vi "Load State Machine.vi"   [LabVIEW 2013]
uses:
  typedefs/fg_typedef.ctl
  typedefs/State Machine/singleUseSubstate.ctl
  <vilib>/Rock Robotics/WPI/Solenoid/WPI_SolenoidValue.ctl
  typedefs/DevRef Type.ctl
  typedefs/State Machine/subStates.ctl
  <vilib>/Rock Robotics/WPI/Solenoid/WPI_SolenoidGetEnum.vi
panel:
  # "A State Machine to Handle Loading for Either High or Low Goal Shots"
types:
  T1 = typedef "fg_typedef.ctl" = enum16{"Get", "Set"}
  T2 = typedef "DevRef Type.ctl" = enum16{"Shooter Solenoid", "Latch Solenoid", "Right Up Sensor", "Right Down Sensor", "Hold Sensor", "2 Ball Switch", "Arm Encoder"}
  T3 = typedef "WPI_SolenoidValue.ctl" = enum16{"Off", "On", "Forward", "Reverse"}
  T4 = typedef "singleUseSubstate.ctl" = enum16{"null", "wait", "shift high", "shift low", "extend shooter", "retract shooter", "latch", "unlatch", "end"}
  T5 = typedef "subStates.ctl" = enum16{"null", "wait", "driver control", "auto", "manual override", "hold position", "rotate", "pickup", "pass", "recover pass", "load", "goto shoot", "shoot high goal", "shoot low goal", "cancel arm", "cancel shooter", "end", "test"}
  T6 = typedef "WPI_SolenoidDevRef.ctl" = cluster{"DevStatus":errorcluster, "Solenoid Module":T7, "Forward Solenoid Channel":T8, "Reverse Solenoid Channel":T8}
  T7 = typedef "FPGA_TypedefSolenoidModule.ctl" = enum16{"Solenoid Module 1", "Solenoid Module 2"}
  T8 = typedef "WPI_SolenoidChannel.ctl" = enum8{"Solenoid 1", "Solenoid 2", "Solenoid 3", "Solenoid 4", "Solenoid 5", "Solenoid 6", "Solenoid 7", "Solenoid 8", "Invalid"}
  T9 = typedef "WPI_DigitalInputDevRef.ctl" = cluster{"DevStatus":errorcluster, "DIO Channel":T10, "Digital Module":T11}
  T10 = typedef "FPGA_DIOChannel.ctl" = enum8{"DIO 1", "DIO 2", "DIO 3", "DIO 4", "DIO 5", "DIO 6", "DIO 7", "DIO 8", "DIO 9", "DIO 10", "DIO 11", "DIO 12", "DIO 13", "DIO 14", "Invalid"}
  T11 = typedef "FPGA_TypedefDigitalModule.ctl" = enum16{"Digital Module 1", "Digital Module 2"}
  T12 = typedef "WPI_EncoderDevRef.ctl" = cluster{"DevStatus":errorcluster, "EncoderIndex":T13, "CounterIndex":T14, "DistancePerCount":dbl, "Decoding Type":T15}
  T13 = typedef "FPGA_EncoderIdx.ctl" = enum8{"Enc 0", "Enc 1", "Enc 2", "Enc 3", "Invalid"}
  T14 = typedef "FPGA_CounterCtrSystemIndex.ctl" = enum8{"Ctr 0", "Ctr 1", "Ctr 2", "Ctr 3", "Ctr 4", "Ctr 5", "Ctr 6", "Ctr 7", "Invalid"}
  T15 = typedef "WPI_EncoderType.ctl" = enum16{"1x", "2x", "4x"}
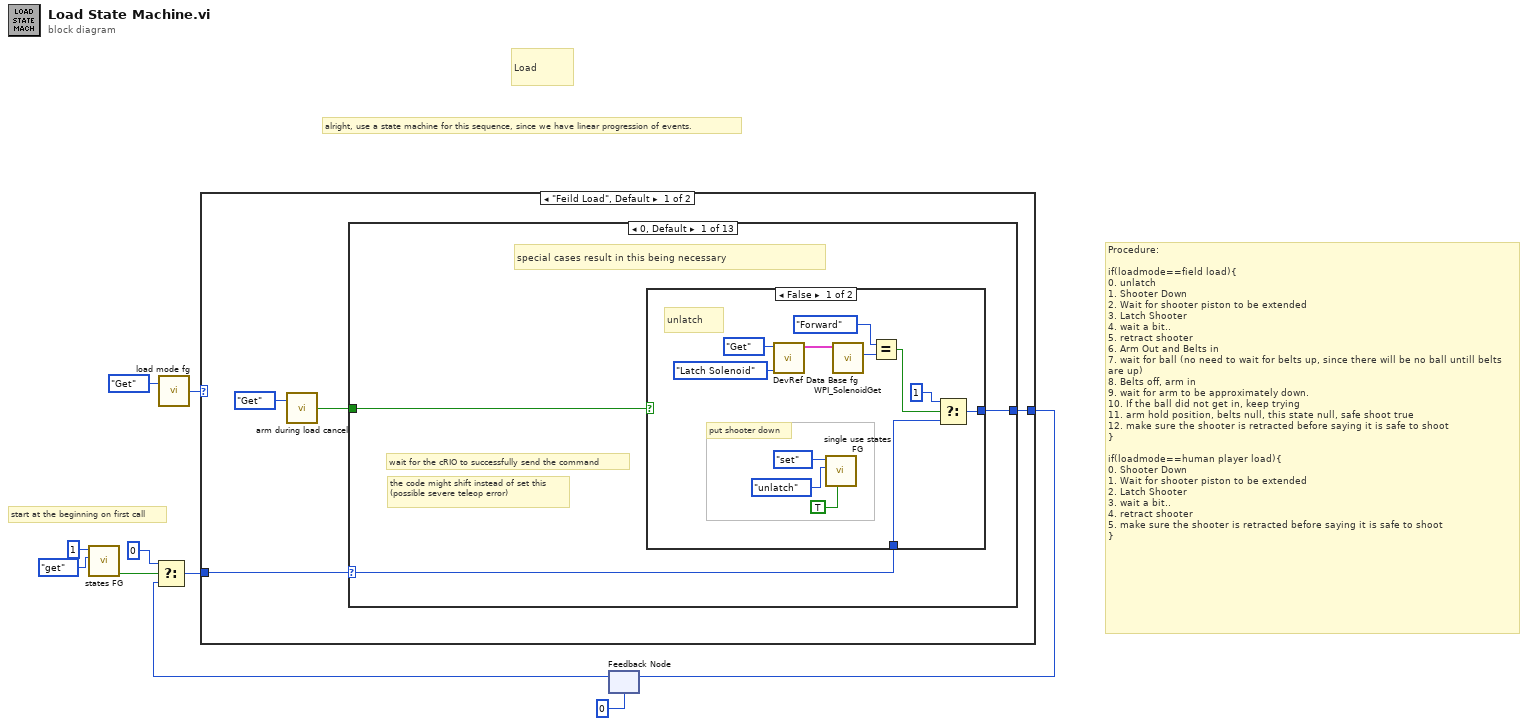
[diagram p0: block diagram]
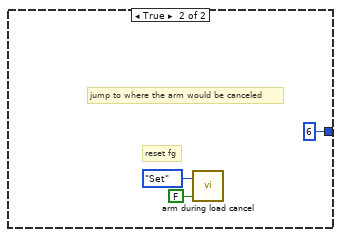
[diagram p2: hidden frame]
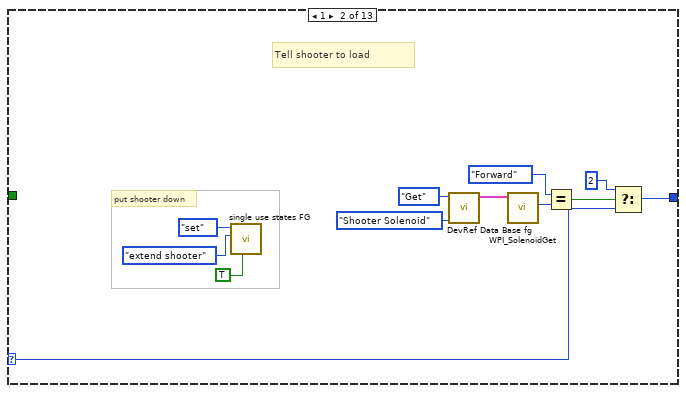
[diagram p3: hidden frame]
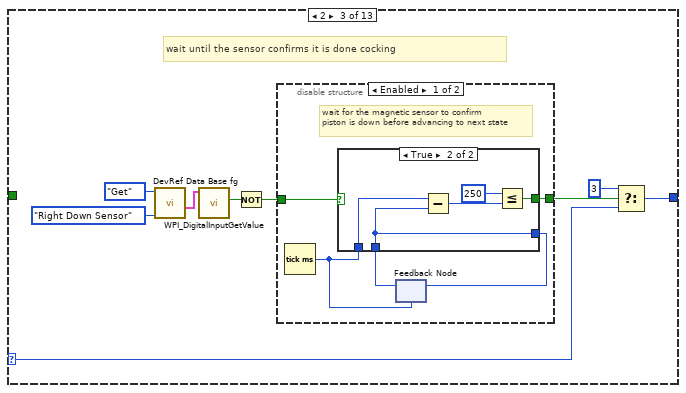
[diagram p4: hidden frame]
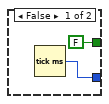
[diagram p5: hidden frame]
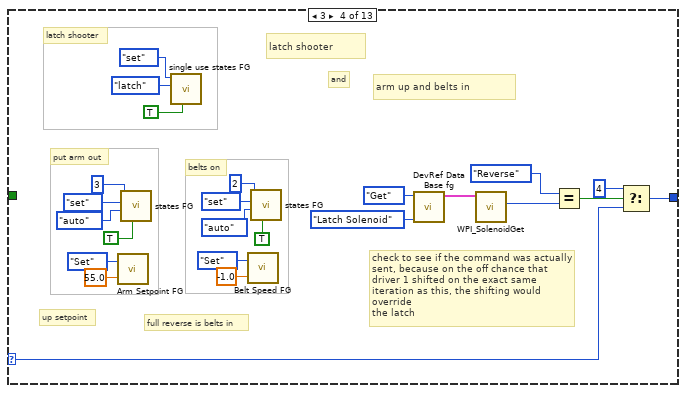
[diagram p7: hidden frame]
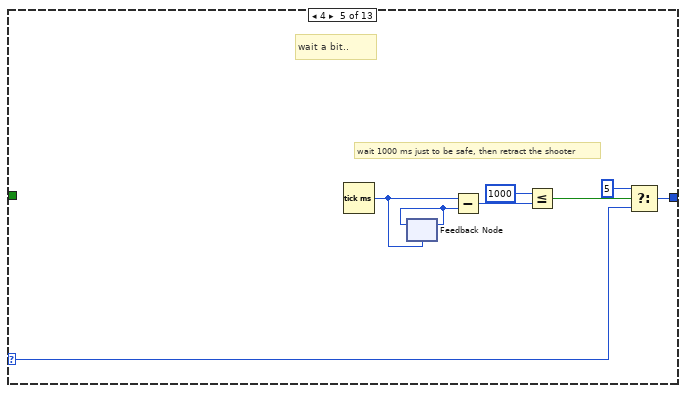
[diagram p8: hidden frame]
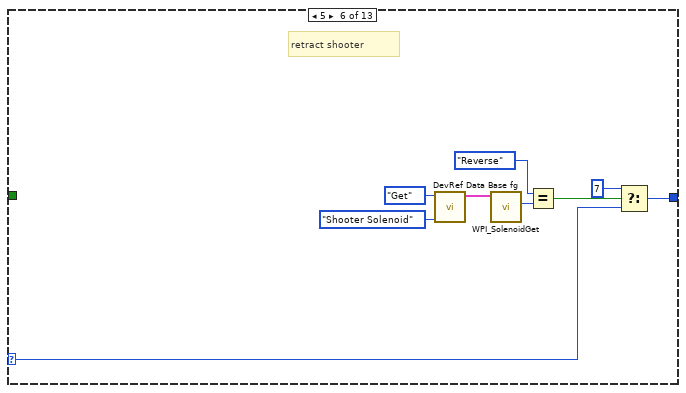
[diagram p9: hidden frame]
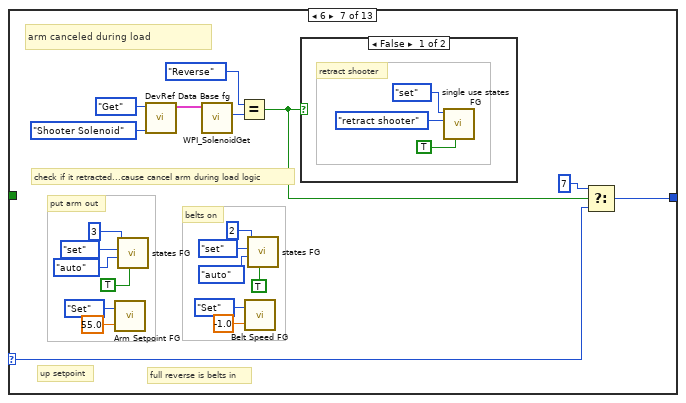
[diagram p10: hidden frame]
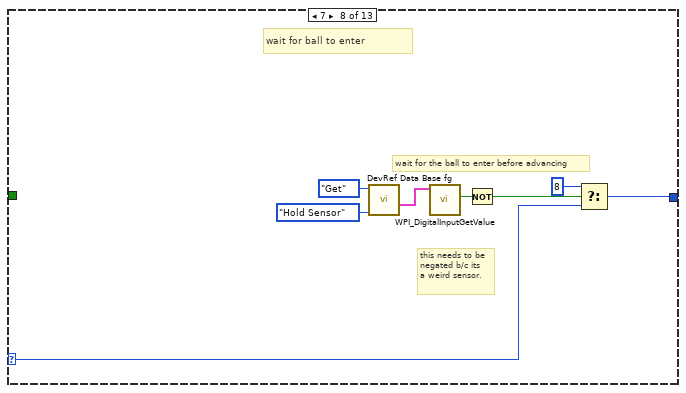
[diagram p12: hidden frame]
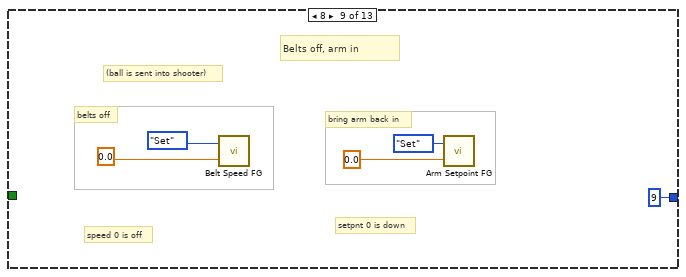
[diagram p13: hidden frame]
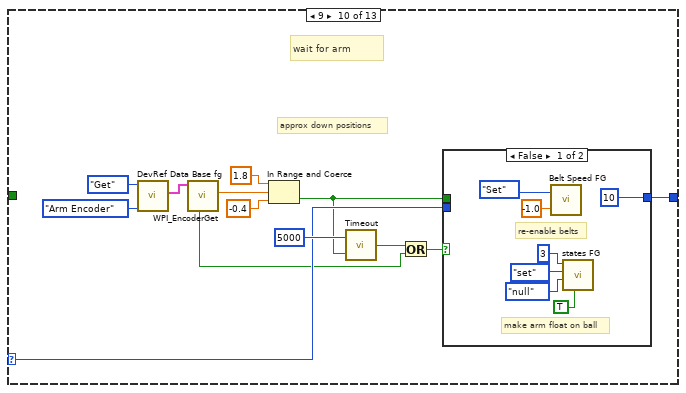
[diagram p14: hidden frame]
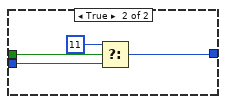
[diagram p15: hidden frame]
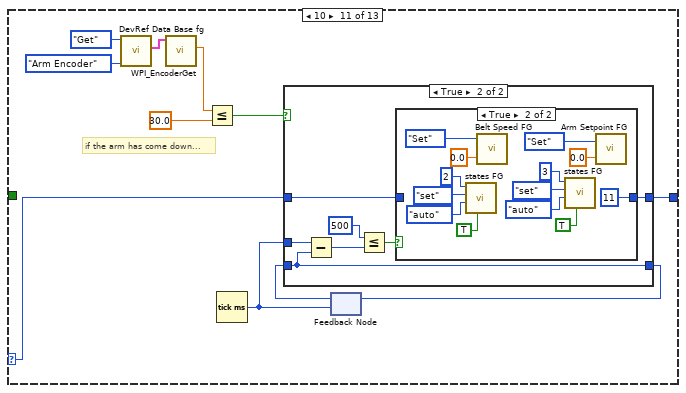
[diagram p16: hidden frame]
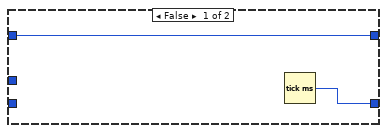
[diagram p17: hidden frame]
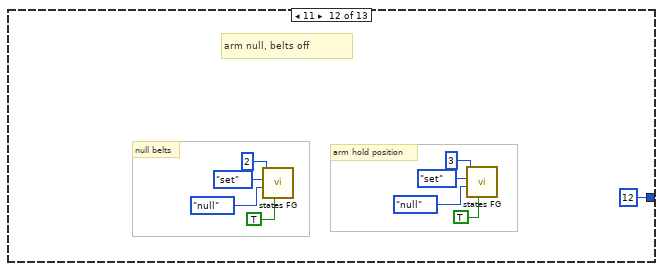
[diagram p19: hidden frame]
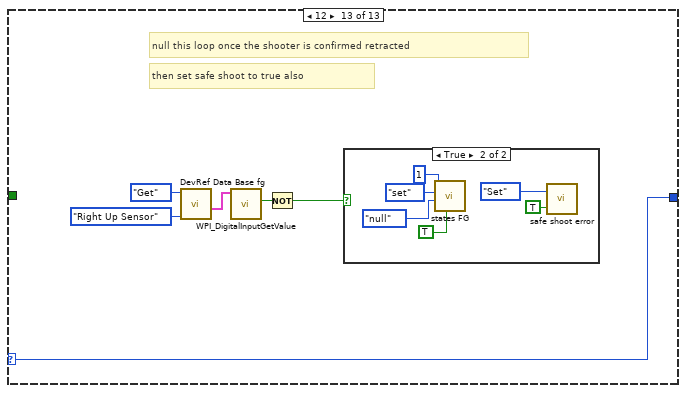
[diagram p20: hidden frame]
diagram:
  # "start at the beginning on first call"
  # "Load"
  # "Procedure: \n\nif(loadmode==field load){\n0. unlatch\n1. Shooter Down \n2. Wait for shooter piston to be extended\n3. Latch Shooter\n4. wait a bit..\n5. retract shooter\n6. Arm Out and Belts in\n7. wait for ball (no need to wait for belts up, since there will be no ball untill belts are up)\n8. Belts off, arm in\n9. wait for arm to be approximately down.\n10. If the ball did not get in, keep trying\n11. arm hold position, belts null, this state null, safe shoot true\n12. make sure the shooter is retracted before saying it is safe to shoot\n}\n\nif(loadmode==human player load){\n0. Shooter Down \n1. Wait for shooter piston to be extended\n2. Latch Shooter\n3. wait a bit..\n4. retract shooter\n5. make sure the shooter is retracted before saying it is safe to shoot\n}"
  # "alright, use a state machine for this sequence, since we have linear progression of events."
  n1 = call "states FG.vi"("menu (get)"=enum16{"set", "get"}."get", "Loop ID"=1) -> ("first call?"=w3:bool)  [unwired: 6 in, 3 out]
  n2 = call "load mode fg.vi"("Menu"=fg_typedef."Get") -> ("Load Mode"=w2:enum16{"Feild Load", "Human Player Load"})  [unwired: 1 in]
  n3 = feedback #1(u8 0) -> (w4:u8)
  n4 = Select(t=u8 0, s=w3, f=w4) -> (s? t:f=w6:u8)
  n5 = case shown="\"Feild Load\", Default" w2 {
    tunnel: [w14 w225] -> w9
    tunnel: w6 -> [w13 w224]
    frame "Feild Load", Default {
      n6 = call "arm during load cancel.vi"("Mode"=enum16{"Get", "Set", "Teleop Set"}."Get") -> ("Arm Canceled During Load"=w11:bool)  [unwired: 1 in]
      n7 = case shown="0, Default" w13 {
        selector: w13 -> [w16 w33 w51 w86 w92 w107 w120 w137 _ w149 w169 _ w217]
        tunnel: [w17 w34 w50 w87 w94 w106 w121 w136 u8 9 ("t") w150 w171 u8 12 ("t") w217] -> w14
        tunnel: w11 -> [w15 _ _ _ _ _ _ _ _ _ _ _ _]
        frame 0, Default {
          # "the code might shift instead of set this\n(possible severe teleop error)"
          # "special cases result in this being necessary"
          # "wait for the cRIO to successfully send the command"
          n8 = case shown="False" w15 {
            tunnel: [w26 u8 6 ("t")] -> w17
            tunnel: w16 -> [w25 _]
            frame False {
              # "unlatch"
              # "put shooter down"
              n9 = call "DevRef Data Base fg.vi"("DevRef to Get"=DevRef_Type."Latch Solenoid", "Menu"=fg_typedef."Get") -> ("Selected Solenoid"=w24:T6)  [unwired: 2 in, 5 out]
              n10 = call "single use states FG.vi"("exit in"=TRUE, "substate"=singleUseSubstate."unlatch", "menu (get)"=enum16{"set", "get"}."set") -> ()  [unwired: 5 in, 4 out]
              n11 = call-poly <vilib>:"WPI_SolenoidGet.vi"("SolenoidDevRef"=w24) -> ("Value"=w23:T3)  [unwired: 8 in, 2 out]
              n12 = Equal?(x=WPI_SolenoidValue."Forward", y=w23) -> (x = y?=w21:bool)
              n13 = Select(t=u8 1, s=w21, f=w25) -> (s? t:f=w26:u8)
            }
            frame True {
              # "reset fg"
              # "jump to where the arm would be canceled"
              n14 = call "arm during load cancel.vi"("Arm Canceled During Load?"=FALSE, "Mode"=enum16{"Get", "Set", "Teleop Set"}."Set") -> ()  [unwired: 1 out]
            }
          }
        }
        frame 1 {
          # "Tell shooter to load"
          # "put shooter down"
          n15 = call "single use states FG.vi"("exit in"=TRUE, "substate"=singleUseSubstate."extend shooter", "menu (get)"=enum16{"set", "get"}."set") -> ()  [unwired: 5 in, 4 out]
          n16 = call "DevRef Data Base fg.vi"("DevRef to Get"=DevRef_Type."Shooter Solenoid", "Menu"=fg_typedef."Get") -> ("Selected Solenoid"=w41:T6)  [unwired: 2 in, 5 out]
          n17 = call-poly <vilib>:"WPI_SolenoidGet.vi"("SolenoidDevRef"=w41) -> ("Value"=w40:T3)  [unwired: 8 in, 2 out]
          n18 = Equal?(x=WPI_SolenoidValue."Forward", y=w40) -> (x = y?=w38:bool)
          n19 = Select(t=u8 2, s=w38, f=w33) -> (s? t:f=w34:u8)
        }
        frame 2 {
          # "wait until the sensor confirms it is done cocking"
          n20 = call "DevRef Data Base fg.vi"("DevRef to Get"=DevRef_Type."Right Down Sensor", "Menu"=fg_typedef."Get") -> ("Selected Sensor"=w52:T9)  [unwired: 2 in, 5 out]
          n21 = call <vilib>:"WPI_DigitalInputGetValue.vi"("DigitalInputDevRef"=w52) -> ("Value"=w53:bool)  [unwired: 8 in, 2 out]
          n22 = Not(x=w53) -> (.not. x?=w46:bool)
          n23 = disable-structure shown="Enabled" {
            disable-tunnel: w46 -> [w58 w66]
            disable-tunnel: [w54 w66] -> w45
            frame Enabled {
              # "wait for the magnetic sensor to confirm \npiston is down before advancing to next state"
              n24 = Tick Count (ms)() -> (millisecond timer value=w57:u32)
              n25 = feedback #2(w57) -> (w55:u32)
              n26 = case shown="True" w58 {
                tunnel: w57 -> [_ w63]
                tunnel: [w60 w61] -> w56
                tunnel: w55 -> [_ w61]
                tunnel: [FALSE w62] -> w54
                frame False {
                  n27 = Tick Count (ms)() -> (millisecond timer value=w60:u32)
                }
                frame True {
                  n28 = Subtract(x=w63, y=w61) -> (x-y=w65:u32)
                  n29 = Less Or Equal?(x=u32 250, y=w65) -> (x <= y?=w62:bool)
                }
              }
              n30 = feedback-in #2(w56) -> ()
            }
            frame Disabled {
            }
          }
          n31 = Select(t=u8 3, s=w45, f=w51) -> (s? t:f=w50:u8)
        }
        frame 3 {
          # "latch shooter"
          # "full reverse is belts in"
          # "belts on"
          # "up setpoint"
          # "put arm out"
          # "and"
          # "arm up and belts in"
          # "check to see if the command was actually\nsent, because on the off chance that\ndriver 1 shifted on the exact same\niteration as this, the shifting would override\nthe latch"
          # "latch shooter"
          n32 = call "Arm Setpoint FG.vi"("Setpoint In"=55.0, "Menu"=fg_typedef."Set") -> ()  [unwired: 1 out]
          n33 = call "states FG.vi"("exit in"=TRUE, "subState in"=subStates."auto", "menu (get)"=enum16{"set", "get"}."set", "Loop ID"=3) -> ()  [unwired: 4 in, 4 out]
          n34 = call "single use states FG.vi"("exit in"=TRUE, "substate"=singleUseSubstate."latch", "menu (get)"=enum16{"set", "get"}."set") -> ()  [unwired: 5 in, 4 out]
          n35 = call "Belt Speed FG.vi"("Speed In"=-1.0 ("Setpoint In"), "Menu"=fg_typedef."Set") -> ()  [unwired: 1 out]
          n36 = call "states FG.vi"("exit in"=TRUE, "subState in"=subStates."auto", "menu (get)"=enum16{"set", "get"}."set", "Loop ID"=2) -> ()  [unwired: 4 in, 4 out]
          n37 = call "DevRef Data Base fg.vi"("DevRef to Get"=DevRef_Type."Latch Solenoid", "Menu"=fg_typedef."Get") -> ("Selected Solenoid"=w85:T6)  [unwired: 2 in, 5 out]
          n38 = call-poly <vilib>:"WPI_SolenoidGet.vi"("SolenoidDevRef"=w85) -> ("Value"=w84:T3)  [unwired: 8 in, 2 out]
          n39 = Equal?(x=WPI_SolenoidValue."Reverse" ("Value"), y=w84) -> (x = y?=w82:bool)
          n40 = Select(t=u8 4, s=w82, f=w86) -> (s? t:f=w87:u8)
        }
        frame 4 {
          # "wait a bit.."
          # "wait 1000 ms just to be safe, then retract the shooter"
          n41 = Tick Count (ms)() -> (millisecond timer value=w96:u32)
          n42 = feedback #3(w96) -> (w97:u32)
          n43 = feedback-in #3(w97) -> ()
          n44 = Subtract(x=w96, y=w97) -> (x-y=w95:u32)
          n45 = Less Or Equal?(x=u32 1000, y=w95) -> (x <= y?=w93:bool)
          n46 = Select(t=u8 5, s=w93, f=w92) -> (s? t:f=w94:u8)
        }
        frame 5 {
          # "retract shooter"
          n47 = call "DevRef Data Base fg.vi"("DevRef to Get"=DevRef_Type."Shooter Solenoid", "Menu"=fg_typedef."Get") -> ("Selected Solenoid"=w105:T6)  [unwired: 2 in, 5 out]
          n48 = call-poly <vilib>:"WPI_SolenoidGet.vi"("SolenoidDevRef"=w105) -> ("Value"=w104:T3)  [unwired: 8 in, 2 out]
          n49 = Equal?(x=WPI_SolenoidValue."Reverse", y=w104) -> (x = y?=w102:bool)
          n50 = Select(t=u8 7, s=w102, f=w107) -> (s? t:f=w106:u8)
        }
        frame 6 {
          # "full reverse is belts in"
          # "belts on"
          # "up setpoint"
          # "put arm out"
          # "check if it retracted...cause cancel arm during load logic"
          # "arm canceled during load"
          n51 = call "Arm Setpoint FG.vi"("Setpoint In"=55.0, "Menu"=fg_typedef."Set") -> ()  [unwired: 1 out]
          n52 = call "states FG.vi"("exit in"=TRUE, "subState in"=subStates."auto", "menu (get)"=enum16{"set", "get"}."set", "Loop ID"=3) -> ()  [unwired: 4 in, 4 out]
          n53 = call "DevRef Data Base fg.vi"("DevRef to Get"=DevRef_Type."Shooter Solenoid", "Menu"=fg_typedef."Get") -> ("Selected Solenoid"=w128:T6)  [unwired: 2 in, 5 out]
          n54 = call-poly <vilib>:"WPI_SolenoidGet.vi"("SolenoidDevRef"=w128) -> ("Value"=w127:T3)  [unwired: 8 in, 2 out]
          n55 = Equal?(x=WPI_SolenoidValue."Reverse", y=w127) -> (x = y?=w122:bool)
          n56 = call "Belt Speed FG.vi"("Speed In"=-1.0 ("Setpoint In"), "Menu"=fg_typedef."Set") -> ()  [unwired: 1 out]
          n57 = call "states FG.vi"("exit in"=TRUE, "subState in"=subStates."auto", "menu (get)"=enum16{"set", "get"}."set", "Loop ID"=2) -> ()  [unwired: 4 in, 4 out]
          n58 = case shown="False" w122 {
            frame False {
              # "retract shooter"
              n59 = call "single use states FG.vi"("exit in"=TRUE, "substate"=singleUseSubstate."retract shooter", "menu (get)"=enum16{"set", "get"}."set") -> ()  [unwired: 5 in, 4 out]
            }
            frame True {
            }
          }
          n60 = Select(t=u8 7, s=w122, f=w120) -> (s? t:f=w121:u8)
        }
        frame 7 {
          # "this needs to be\nnegated b/c its\na weird sensor."
          # "wait for the ball to enter before advancing"
          # "wait for ball to enter"
          n61 = call "DevRef Data Base fg.vi"("DevRef to Get"=DevRef_Type."Hold Sensor", "Menu"=fg_typedef."Get") -> ("Selected Sensor"=w135:T9)  [unwired: 2 in, 5 out]
          n62 = call <vilib>:"WPI_DigitalInputGetValue.vi"("DigitalInputDevRef"=w135) -> ("Value"=w139:bool)  [unwired: 8 in, 2 out]
          n63 = Not(x=w139) -> (.not. x?=w138:bool)
          n64 = Select(t=u8 8, s=w138, f=w137) -> (s? t:f=w136:u8)
        }
        frame 8 {
          # "bring arm back in"
          # "setpnt 0 is down"
          # "speed 0 is off"
          # "Belts off, arm in"
          # "(ball is sent into shooter)"
          # "belts off"
          n65 = call "Belt Speed FG.vi"("Speed In"=0.0 ("Setpoint In"), "Menu"=fg_typedef."Set") -> ()  [unwired: 1 out]
          n66 = call "Arm Setpoint FG.vi"("Setpoint In"=0.0, "Menu"=fg_typedef."Set") -> ()  [unwired: 1 out]
        }
        frame 9 {
          # "approx down positions"
          # "wait for arm"
          n67 = call "DevRef Data Base fg.vi"("DevRef to Get"=DevRef_Type."Arm Encoder", "Menu"=fg_typedef."Get") -> ("Selected Encoder"=w157:T12)  [unwired: 2 in, 5 out]
          n68 = call <vilib>:"WPI_EncoderGet.vi"("EncoderDevRef"=w157) -> ("Distance"=w156:dbl, "Stopped"=w145:bool)  [unwired: 5 in, 4 out]
          n69 = In Range and Coerce(upper limit=1.8, x=w156, lower limit=-0.4) -> (In Range?=w148:bool)  [unwired: 1 out]
          n70 = call "Timeout.vi"("Done with Task?"=w148, "Timeout (ms)"=u32 5000) -> ("Timed Out?"=w146:bool)  [unwired: 1 in]
          n71 = Or(x=w146, y=w145) -> (x .or. y?=w147:bool)
          n72 = case shown="False" w147 {
            tunnel: w149 -> [_ w168]
            tunnel: [u8 10 ("t") w167] -> w150
            tunnel: w148 -> [_ w165]
            frame False {
              # "re-enable belts"
              # "make arm float on ball"
              n73 = call "Belt Speed FG.vi"("Speed In"=-1.0, "Menu"=fg_typedef."Set") -> ()  [unwired: 1 out]
              n74 = call "states FG.vi"("exit in"=TRUE, "subState in"=subStates."null", "menu (get)"=enum16{"set", "get"}."set", "Loop ID"=3) -> ()  [unwired: 4 in, 4 out]
            }
            frame True {
              n75 = Select(t=u8 11, s=w165, f=w168) -> (s? t:f=w167:u8)
            }
          }
        }
        frame 10 {
          # "if the arm has come down..."
          n76 = call "DevRef Data Base fg.vi"("DevRef to Get"=DevRef_Type."Arm Encoder", "Menu"=fg_typedef."Get") -> ("Selected Encoder"=w175:T12)  [unwired: 2 in, 5 out]
          n77 = call <vilib>:"WPI_EncoderGet.vi"("EncoderDevRef"=w175) -> ("Distance"=w179:dbl)  [unwired: 5 in, 5 out]
          n78 = Less Or Equal?(x=w179, y=30.0) -> (x <= y?=w170:bool)
          n79 = Tick Count (ms)() -> (millisecond timer value=w173:u32)
          n80 = feedback #4(w173) -> (w174:u32)
          n81 = case shown="True" w170 {
            tunnel: [w181 w188] -> w172
            tunnel: w174 -> [_ w188]
            tunnel: w173 -> [_ w187]
            tunnel: [w180 w183] -> w171
            tunnel: w169 -> [w180 w182]
            frame False {
              n82 = Tick Count (ms)() -> (millisecond timer value=w181:u32)
            }
            frame True {
              n83 = Subtract(x=w187, y=w188) -> (x-y=w186:u32)
              n84 = Less Or Equal?(x=u32 500, y=w186) -> (x <= y?=w184:bool)
              n85 = case shown="True" w184 {
                tunnel: [w189 u8 11] -> w183
                tunnel: w182 -> [w189 _]
                frame False {
                }
                frame True {
                  n86 = call "states FG.vi"("exit in"=TRUE, "subState in"=subStates."auto", "menu (get)"=enum16{"set", "get"}."set", "Loop ID"=2) -> ()  [unwired: 4 in, 4 out]
                  n87 = call "Belt Speed FG.vi"("Speed In"=0.0, "Menu"=fg_typedef."Set") -> ()  [unwired: 1 out]
                  n88 = call "states FG.vi"("exit in"=TRUE, "subState in"=subStates."auto", "menu (get)"=enum16{"set", "get"}."set", "Loop ID"=3) -> ()  [unwired: 4 in, 4 out]
                  n89 = call "Arm Setpoint FG.vi"("Setpoint In"=0.0, "Menu"=fg_typedef."Set") -> ()  [unwired: 1 out]
                }
              }
            }
          }
          n90 = feedback-in #4(w172) -> ()
        }
        frame 11 {
          # "null belts"
          # "arm null, belts off"
          # "arm hold position"
          n91 = call "states FG.vi"("exit in"=TRUE, "subState in"=subStates."null", "menu (get)"=enum16{"set", "get"}."set", "Loop ID"=2) -> ()  [unwired: 4 in, 4 out]
          n92 = call "states FG.vi"("exit in"=TRUE, "subState in"=subStates."null", "menu (get)"=enum16{"set", "get"}."set", "Loop ID"=3) -> ()  [unwired: 4 in, 4 out]
        }
        frame 12 {
          # "then set safe shoot to true also"
          # "null this loop once the shooter is confirmed retracted"
          n93 = call "DevRef Data Base fg.vi"("DevRef to Get"=DevRef_Type."Right Up Sensor", "Menu"=fg_typedef."Get") -> ("Selected Sensor"=w216:T9)  [unwired: 2 in, 5 out]
          n94 = call <vilib>:"WPI_DigitalInputGetValue.vi"("DigitalInputDevRef"=w216) -> ("Value"=w215:bool)  [unwired: 8 in, 2 out]
          n95 = Not(x=w215) -> (.not. x?=w214:bool)
          n96 = case shown="True" w214 {
            frame False {
            }
            frame True {
              n97 = call "states FG.vi"("exit in"=TRUE, "subState in"=subStates."null", "menu (get)"=enum16{"set", "get"}."set", "Loop ID"=1) -> ()  [unwired: 4 in, 4 out]
              n98 = call "safe shoot error.vi"("Can Shoot Safely?"=TRUE, "Menu"=fg_typedef."Set") -> ()  [unwired: 1 out]
            }
          }
        }
      }
    }
    frame "Human Player Load" {
      n99 = case shown="0, Default" w224 {
        selector: w224 -> [w226 w248 w257 w279 w285 w300 w311]
        tunnel: [w227 w249 w256 w280 w287 w299 w311] -> w225
        frame 0, Default {
          # "put shooter down"
          # "since that has caused probelms not having this"
          # "unlatch"
          n100 = call "single use states FG.vi"("exit in"=TRUE, "substate"=singleUseSubstate."unlatch", "menu (get)"=enum16{"set", "get"}."set") -> ()  [unwired: 5 in, 4 out]
          n101 = call "DevRef Data Base fg.vi"("DevRef to Get"=DevRef_Type."Latch Solenoid", "Menu"=fg_typedef."Get") -> ("Selected Solenoid"=w234:T6)  [unwired: 2 in, 5 out]
          n102 = call-poly <vilib>:"WPI_SolenoidGet.vi"("SolenoidDevRef"=w234) -> ("Value"=w233:T3)  [unwired: 8 in, 2 out]
          n103 = Equal?(x=WPI_SolenoidValue."Forward", y=w233) -> (x = y?=w231:bool)
          n104 = Select(t=u8 1, s=w231, f=w226) -> (s? t:f=w227:u8)
        }
        frame 1 {
          # "put shooter down"
          # "Wait for shooter to be cocked"
          # "Tell shooter to load"
          n105 = call "single use states FG.vi"("exit in"=TRUE, "substate"=singleUseSubstate."extend shooter", "menu (get)"=enum16{"set", "get"}."set") -> ()  [unwired: 5 in, 4 out]
          n106 = call "DevRef Data Base fg.vi"("DevRef to Get"=DevRef_Type."Shooter Solenoid", "Menu"=fg_typedef."Get") -> ("Selected Solenoid"=w244:T6)  [unwired: 2 in, 5 out]
          n107 = call-poly <vilib>:"WPI_SolenoidGet.vi"("SolenoidDevRef"=w244) -> ("Value"=w243:T3)  [unwired: 8 in, 2 out]
          n108 = Equal?(x=WPI_SolenoidValue."Forward", y=w243) -> (x = y?=w241:bool)
          n109 = Select(t=u8 2, s=w241, f=w248) -> (s? t:f=w249:u8)
        }
        frame 2 {
          # "wait for the magnetic sensor to confirm \npiston is down before advancing to next state"
          # "wait until the sensor confirms it is done cocking"
          n110 = call "DevRef Data Base fg.vi"("DevRef to Get"=DevRef_Type."Right Down Sensor", "Menu"=fg_typedef."Get") -> ("Selected Sensor"=w258:T9)  [unwired: 2 in, 5 out]
          n111 = call <vilib>:"WPI_DigitalInputGetValue.vi"("DigitalInputDevRef"=w258) -> ("Value"=w251:bool)  [unwired: 8 in, 2 out]
          n112 = Not(x=w251) -> (.not. x?=w252:bool)
          n113 = disable-structure shown="Enabled" {
            disable-tunnel: w252 -> [w263 w271]
            disable-tunnel: [w259 w271] -> w250
            frame Enabled {
              n114 = Tick Count (ms)() -> (millisecond timer value=w262:u32)
              n115 = feedback #5(w262) -> (w260:u32)
              n116 = case shown="True" w263 {
                tunnel: w262 -> [_ w268]
                tunnel: [w265 w266] -> w261
                tunnel: w260 -> [_ w266]
                tunnel: [FALSE w267] -> w259
                frame False {
                  n117 = Tick Count (ms)() -> (millisecond timer value=w265:u32)
                }
                frame True {
                  n118 = Subtract(x=w268, y=w266) -> (x-y=w270:u32)
                  n119 = Less Or Equal?(x=u32 250, y=w270) -> (x <= y?=w267:bool)
                }
              }
              n120 = feedback-in #5(w261) -> ()
            }
            frame Disabled {
            }
          }
          n121 = Select(t=u8 3, s=w250, f=w257) -> (s? t:f=w256:u8)
        }
        frame 3 {
          # "latch shooter"
          # "check to see if the command was actually\nsent, because on the off chance that\ndriver 1 shifted on the exact same\niteration as this, the shifting would override\nthe latch (applies to all instances of this type\nof code logic)"
          # "latch shooter"
          n122 = call "single use states FG.vi"("exit in"=TRUE, "substate"=singleUseSubstate."latch", "menu (get)"=enum16{"set", "get"}."set") -> ()  [unwired: 5 in, 4 out]
          n123 = call "DevRef Data Base fg.vi"("DevRef to Get"=DevRef_Type."Latch Solenoid", "Menu"=fg_typedef."Get") -> ("Selected Solenoid"=w278:T6)  [unwired: 2 in, 5 out]
          n124 = call-poly <vilib>:"WPI_SolenoidGet.vi"("SolenoidDevRef"=w278) -> ("Value"=w277:T3)  [unwired: 8 in, 2 out]
          n125 = Equal?(x=WPI_SolenoidValue."Reverse" ("Value"), y=w277) -> (x = y?=w275:bool)
          n126 = Select(t=u8 4, s=w275, f=w279) -> (s? t:f=w280:u8)
        }
        frame 4 {
          # "wait a bit.."
          # "wait 1000 ms just to be safe, then retract the shooter"
          n127 = Tick Count (ms)() -> (millisecond timer value=w289:u32)
          n128 = feedback #6(w289) -> (w290:u32)
          n129 = feedback-in #6(w290) -> ()
          n130 = Subtract(x=w289, y=w290) -> (x-y=w288:u32)
          n131 = Less Or Equal?(x=u32 1000, y=w288) -> (x <= y?=w286:bool)
          n132 = Select(t=u8 5, s=w286, f=w285) -> (s? t:f=w287:u8)
        }
        frame 5 {
          # "retract shooter"
          # "retract shooter"
          n133 = call "single use states FG.vi"("exit in"=TRUE, "substate"=singleUseSubstate."retract shooter", "menu (get)"=enum16{"set", "get"}."set") -> ()  [unwired: 5 in, 4 out]
          n134 = call "DevRef Data Base fg.vi"("DevRef to Get"=DevRef_Type."Shooter Solenoid", "Menu"=fg_typedef."Get") -> ("Selected Solenoid"=w298:T6)  [unwired: 2 in, 5 out]
          n135 = call-poly <vilib>:"WPI_SolenoidGet.vi"("SolenoidDevRef"=w298) -> ("Value"=w297:T3)  [unwired: 8 in, 2 out]
          n136 = Equal?(x=WPI_SolenoidValue."Reverse", y=w297) -> (x = y?=w295:bool)
          n137 = Select(t=u8 6, s=w295, f=w300) -> (s? t:f=w299:u8)
        }
        frame 6 {
          # "set this false here because it is never\nsupposed to be hit during this type of load\nsince the arm is not used"
          # "then set safe shoot to true also"
          # "null this loop once the shooter is confirmed retracted"
          n138 = call "arm during load cancel.vi"("Arm Canceled During Load?"=FALSE, "Mode"=enum16{"Get", "Set", "Teleop Set"}."Set") -> ()  [unwired: 1 out]
          n139 = call "DevRef Data Base fg.vi"("DevRef to Get"=DevRef_Type."Right Up Sensor", "Menu"=fg_typedef."Get") -> ("Selected Sensor"=w310:T9)  [unwired: 2 in, 5 out]
          n140 = call <vilib>:"WPI_DigitalInputGetValue.vi"("DigitalInputDevRef"=w310) -> ("Value"=w309:bool)  [unwired: 8 in, 2 out]
          n141 = Not(x=w309) -> (.not. x?=w308:bool)
          n142 = case shown="True" w308 {
            frame False {
            }
            frame True {
              n143 = call "states FG.vi"("exit in"=TRUE, "subState in"=subStates."null", "menu (get)"=enum16{"set", "get"}."set", "Loop ID"=1) -> ()  [unwired: 4 in, 4 out]
              n144 = call "safe shoot error.vi"("Can Shoot Safely?"=TRUE, "Menu"=fg_typedef."Set") -> ()  [unwired: 1 out]
            }
          }
        }
      }
    }
  }
  n145 = feedback-in #1(w9) -> ()
